vi "Stop Core.vi"(10 "final error code":i32, 11 "Interface with menu in":refnum<class "Interface with menu.lvclass">) -> (3 "Interface with menu out":refnum<class "Interface with menu.lvclass">)   [LabVIEW 2015, in "Interface with menu.lvclass"]
uses:
  Interface with menu.lvclass
  Interface with menu.lvclass/Interface with menu.ctl
  Mag Lab Measure UI.lvclass
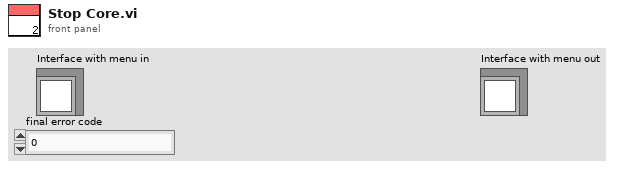
[diagram p1: front panel]
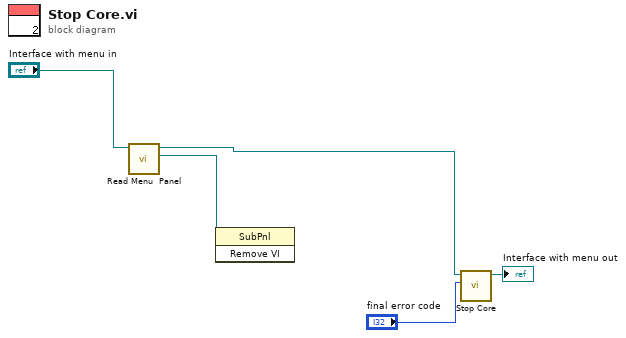
[diagram p0: block diagram]
diagram:
  n1 = call "Read Menu  Panel.vi"("Interface with menu in"="Interface with menu in") -> ("Menu  Panel"=w2:refnum<vi>, "Interface with menu out"=w1:refnum<class "Interface with menu.lvclass">)  [unwired: 8 in, 1 out]
  n2 = invoke class="SubPnl" method="Remove VI"(reference=w2) -> ()  [unwired: 2 in, 3 out]
  n3 = call-parent "Stop Core.vi"("final error code"="final error code", "Mag Lab Measure Interface in"=w1) -> ("Mag Lab Measure Interface out"=→"Interface with menu out":refnum<class "Interface with menu.lvclass">)  [unwired: 9 in]
